vi "Funcion_Apertura_B.vi"(11 "error in (no error)":errorcluster) -> (1 "PIPES":cluster{"PIPE_IN":i32, "PIPE_OUT":i32}, 2 "NDISPOSITIVOS":i32, 3 "error out":errorcluster)   [LabVIEW 2016]
uses:
  <vilib>/Utility/error.llb/Error Cluster From Error Code.vi
  <vilib>/ErrorRing/Error Ring.xnode
  microchip_solutions_v2013-06-15/USB/Tools/MCHPUSB Custom Driver/Mpusbapi/Dll/Borland_C/mpusbapi.dll
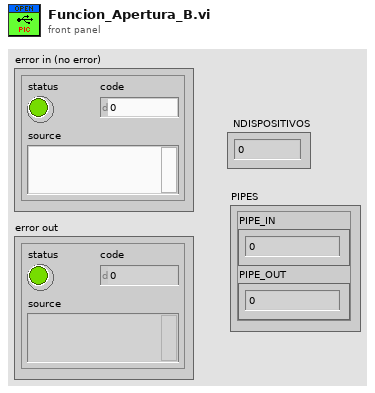
[diagram p1: front panel]
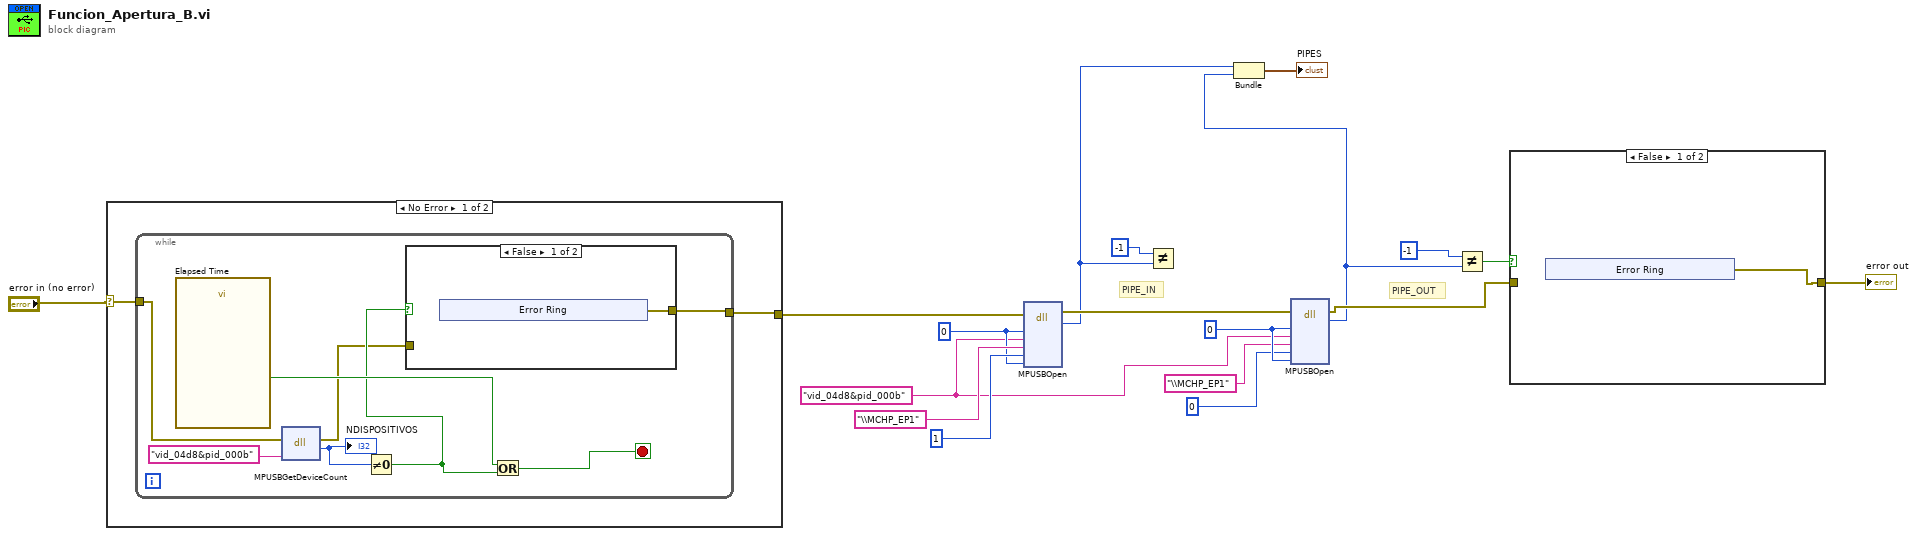
[diagram p0: block diagram]
diagram:
  w1 = "vid_04d8&pid_000b" ("VID_PID")
  w13 = 0 ("Instancia")
  w15 = 0 ("Instancia")
  # "PIPE_OUT"
  # "PIPE_IN"
  n1 = case shown="No Error" "error in (no error)" {
    selector: "error in (no error)" -> [w20 w36]
    tunnel: [w19 w36] -> w14
    frame No Error {
      n2 = while {
        tunnel: w20 -> [w24]
        tunnel: [w23] -> w19
        stop <- w26 stop-if-true
        n3 = call "Elapsed Time"() -> ("Time has Elapsed"=w27:bool)  [unwired: 12 in, 7 out]
        n4 = dll-call lib="C:/microchip_solutions_v2013-06-15/USB/Tools/MCHPUSB Custom Driver/Mpusbapi/Dll/Borland_C/mpusbapi.dll" fn="MPUSBGetDeviceCount"(error in=w24, "VID_PID"="vid_04d8&pid_000b") -> (error out=w21:errorcluster, "NDISPOSITIVOS"=w28:i32)  [unwired: 3 in, 1 out]
        "NDISPOSITIVOS" <- w28
        n5 = Not Equal To 0?(x=w28) -> (x != 0?=w25:bool)
        n6 = case shown="False" w25 {
          tunnel: [w29 w35] -> w23
          tunnel: w21 -> [_ w35]
          frame False {
            n7 = xnode "Error Ring"() -> ("error out"=w29:errorcluster)
          }
          frame True {
          }
        }
        n8 = Or(x=w27, y=w25) -> (x .or. y?=w26:bool)
      }
    }
    frame Error {
    }
  }
  n9 = dll-call lib="C:/microchip_solutions_v2013-06-15/USB/Tools/MCHPUSB Custom Driver/Mpusbapi/Dll/Borland_C/mpusbapi.dll" fn="MPUSBOpen"(error in=w14, "Instancia"=w15, "VID_PID"=w1, "pEP"="\\MCHP_EP1", "dwDIR"=1, "dwReserved"=w15) -> (error out=w10:errorcluster, "PIPE"=w5:i32)  [unwired: 7 in, 1 out]
  n10 = Not Equal?(x=-1, y=w5) -> ()  [unwired: 1 out]
  n11 = dll-call lib="C:/microchip_solutions_v2013-06-15/USB/Tools/MCHPUSB Custom Driver/Mpusbapi/Dll/Borland_C/mpusbapi.dll" fn="MPUSBOpen"(error in=w10, "Instancia"=w13, "VID_PID"=w1, "pEP"="\\MCHP_EP1", "dwDIR"=0, "dwReserved"=w13) -> (error out=w6:errorcluster, "PIPE"=w4:i32)  [unwired: 7 in, 1 out]
  n12 = Bundle("PIPE"=w5, "PIPE"=w4) -> (→"PIPES":cluster{"PIPE":i32, "PIPE":i32})  [unwired: 1 in]
  n13 = Not Equal?(x=-1, y=w4) -> (x != y?=w7:bool)
  n14 = case shown="False" w7 {
    tunnel: w6 -> [_ w43]
    tunnel: [w37 w43] -> w2
    frame False {
      n15 = xnode "Error Ring"() -> ("error out"=w37:errorcluster)
    }
    frame True {
    }
  }
  "error out" <- w2
